vi "Modbus MFC Example.vi"() -> ()   [LabVIEW 2011]
doc: "This VI is an example program of how to use the MKS Modbus Drivers. This VI is only intended to demonstrate the drivers and is not meant to be used as a diagnostic tool."
uses:
  Type Definitions/Modbus Action.ctl
panel:
  out "Valve Drive(%)":sgl min=0 step=1 format="%.1f"
  out "MFC Info":T1
  in  "Flow Zero":bool
  in  "Valve Override":enum32{"Normal", "Close", "Open"}(radio)
  in  "Setpoint":dbl caption="Setpoint(sccm)" min=0.0 step=1.0 format="%#.6g"
  in  "Stop":bool
  in  "Close MB":bool
  in  "Initialize":bool
  in  "MFC IP Address":string="192.168.2.155"
  out "Waveform Chart":cluster{"Flow(sccm)":sgl, "Setpoint":sgl}(graph)
  # "Modbus MFC Example"
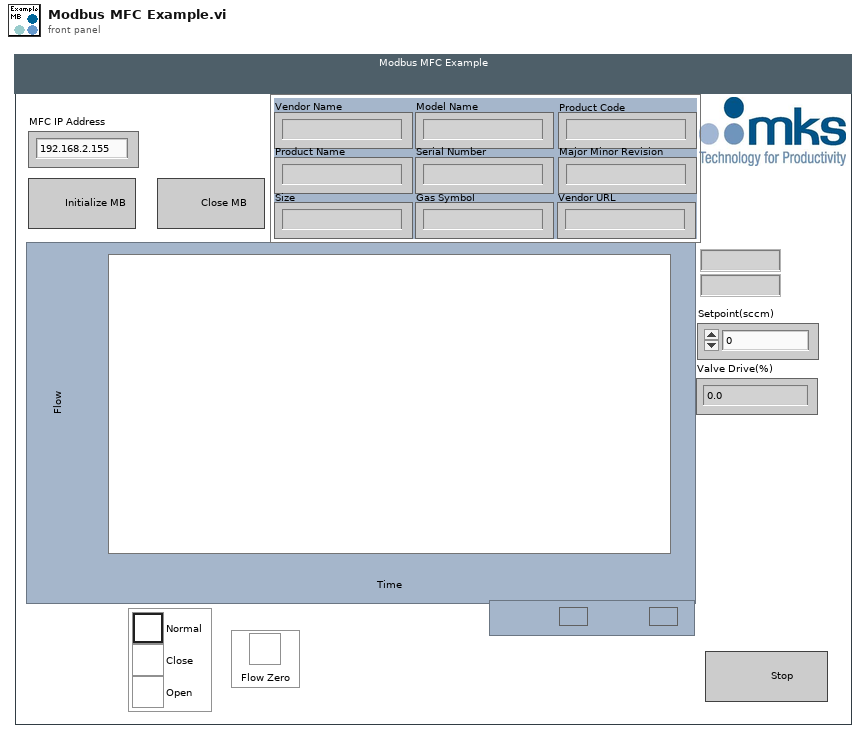
[diagram p1: front panel]
types:
  T1 = cluster{"Vendor Name":string, "Product Code":string, "Major Minor Revision":string, "Vendor URL":string, "Product Name":string, "Model Name":string, "Gas Symbol":string, "Serial Number":string, "Size":string}
  T2 = typedef "Modbus Action.ctl" = enum16{"Read", "Write"}
  T3 = enum8{"Enabled", "Disabled", "Disabled and Grayed Out"}
  T4 = typedef "Valve Override.ctl" = enum16{"Normal", "Close", "Open"}
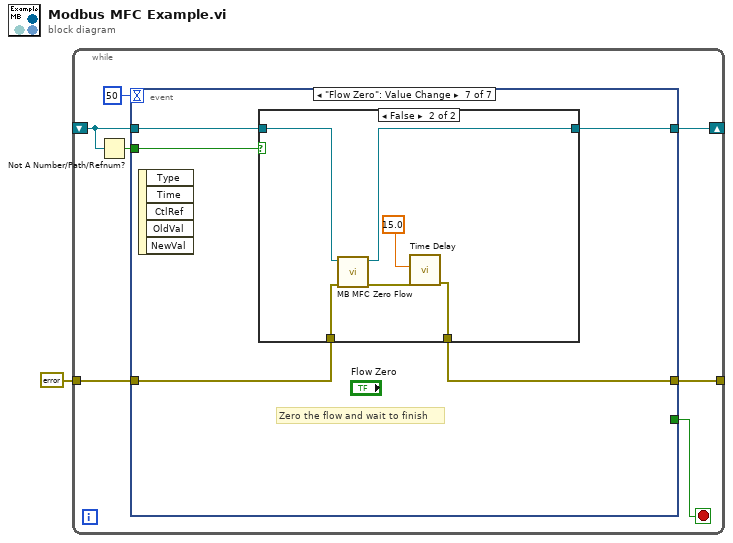
[diagram p0: block diagram]
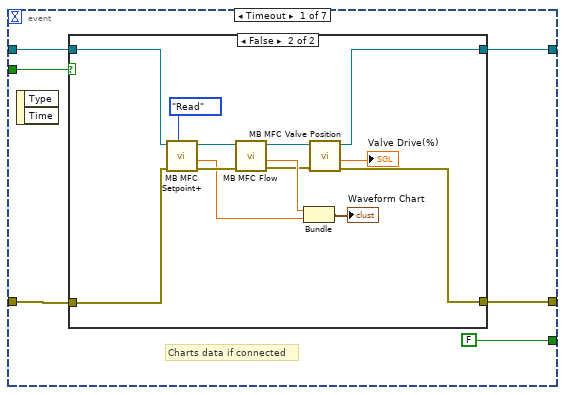
[diagram p2: hidden frame]
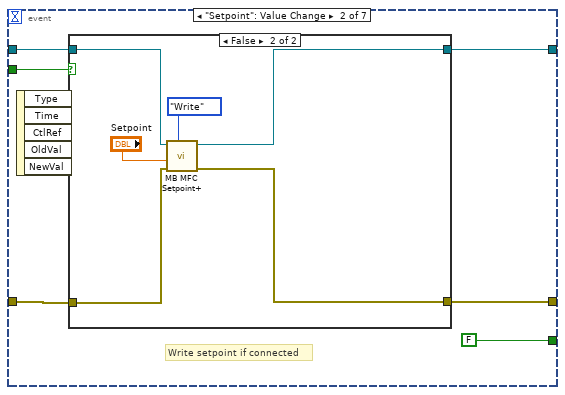
[diagram p4: hidden frame]
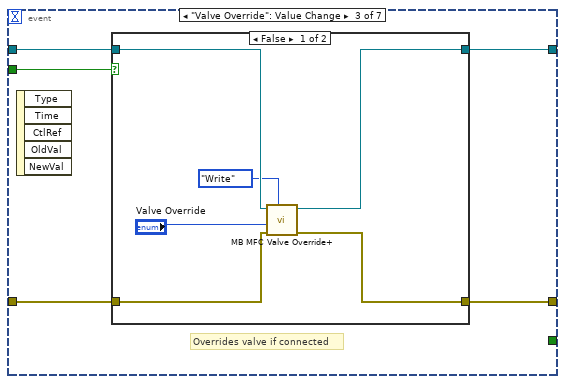
[diagram p6: hidden frame]
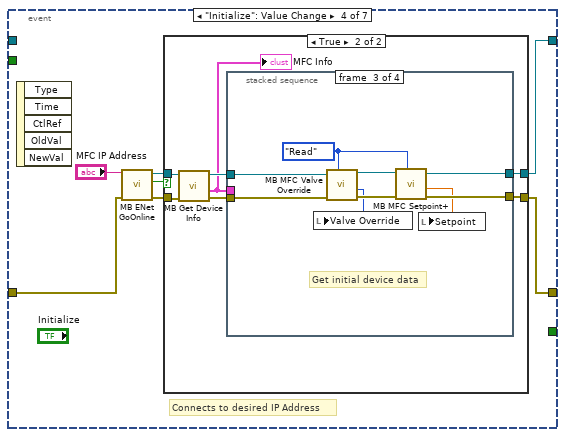
[diagram p8: hidden frame]
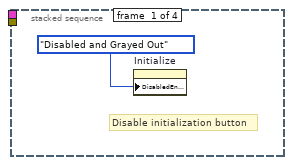
[diagram p10: hidden frame]
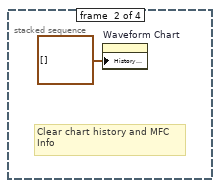
[diagram p11: hidden frame]
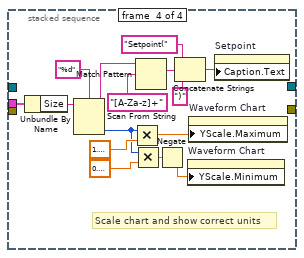
[diagram p12: hidden frame]
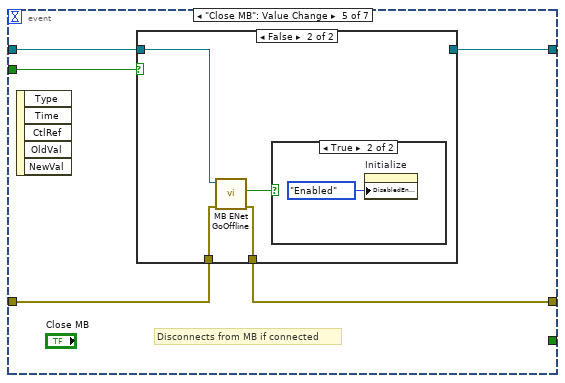
[diagram p13: hidden frame]
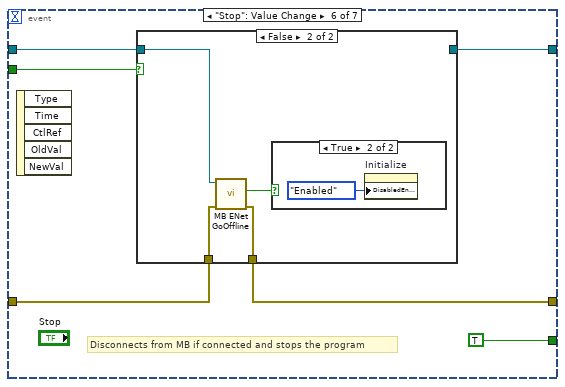
[diagram p16: hidden frame]
diagram:
  n1 = while {
    shift-right: [w6] -> _
    shift-left: _ -> [w3]
    tunnel: errorcluster {"status"=FALSE, "code"=0, "source"=""} ("error out") -> [w5]
    tunnel: [w4] -> _
    stop <- w7 stop-if-true
    n2 = Not A Number/Path/Refnum?(number/path/refnum=w3) -> (NaN/Path/Refnum?=w2:bool)
    n3 = event shown="[6] \"Flow Zero\": Value Change" {
      selector: _ -> [_ _ _ _ _ _ _]
      dyn-events: _ -> [_ _ _ _ _ _ _]
      timeout: 50 -> [_ _ _ _ _ _ _]
      tunnel: [FALSE FALSE _ _ _ TRUE _] -> w7
      tunnel: w3 -> [w10 w31 w48 _ w100 w113 w125]
      tunnel: [w11 w32 w47 w57 w99 w112 w124] -> w6
      tunnel: w5 -> [w13 w34 w45 w62 w102 w115 w127]
      tunnel: [w12 w33 w46 w58 w103 w116 w128] -> w4
      tunnel: w2 -> [w9 w30 w44 _ w101 w114 w126]
      event Timeout {
        # "Charts data if connected"
        n4 = event-data() -> ()  [unwired: 1 in, 2 out]
        n5 = case shown="False" w9 {
          tunnel: w10 -> [w16 w29]
          tunnel: w13 -> [w15 w27]
          tunnel: [w15 w18] -> w12
          tunnel: [w16 w20] -> w11
          frame True {
          }
          frame False {
            n6 = call "MB MFC Setpoint+.vi"("Action"=Modbus_Action."Read", "error in (no error)"=w27, "TCP Ref"=w29) -> ("error out"=w28:errorcluster, "Setpoint"=w24:sgl, "dup TCP Ref"=w26:refnum<k5>)  [unwired: 6 in]
            n7 = call "MB MFC Flow.vi"("error in (no error)"=w28, "TCP Ref"=w26) -> ("error out"=w19:errorcluster, "Flow(sccm)"=w25:sgl, "dup TCP Ref"=w21:refnum<k5>)  [unwired: 7 in]
            n8 = Bundle("Flow(sccm)"=w25, "Setpoint"=w24) -> (→"Waveform Chart":cluster{"Flow(sccm)":sgl, "Setpoint":sgl})  [unwired: 1 in]
            n9 = call "MB MFC Valve Position.vi"("error in (no error)"=w19, "TCP Ref"=w21) -> ("error out"=w18:errorcluster, "Valve Position(%)"=→"Valve Drive(%)":sgl, "dup TCP Ref"=w20:refnum<k5>)  [unwired: 7 in]
          }
        }
      }
      event "Setpoint": Value Change {
        # "Write setpoint if connected"
        n10 = event-data() -> ()  [unwired: 1 in, 5 out]
        n11 = case shown="False" w30 {
          tunnel: w31 -> [w37 w43]
          tunnel: w34 -> [w36 w42]
          tunnel: [w36 w38] -> w33
          tunnel: [w37 w39] -> w32
          frame True {
          }
          frame False {
            n12 = call "MB MFC Setpoint+.vi"("Action"=Modbus_Action."Write", "error in (no error)"=w42, "Setpoint"="Setpoint", "TCP Ref"=w43) -> ("error out"=w38:errorcluster, "dup TCP Ref"=w39:refnum<k5>)  [unwired: 5 in, 1 out]
          }
        }
      }
      event "Valve Override": Value Change {
        # "Overrides valve if connected"
        n13 = event-data() -> ()  [unwired: 1 in, 5 out]
        n14 = case shown="False" w44 {
          tunnel: w48 -> [w53 w55]
          tunnel: [w50 w55] -> w47
          tunnel: [w51 w56] -> w46
          tunnel: w45 -> [w54 w56]
          frame False {
            n15 = call "MB MFC Valve Override+.vi"("Action"=Modbus_Action."Write", "error in (no error)"=w54, "Override"="Valve Override", "TCP Ref"=w53) -> ("error out"=w51:errorcluster, "dup TCP Ref"=w50:refnum<k5>)  [unwired: 5 in, 1 out]
          }
          frame True {
          }
        }
      }
      event "Initialize": Value Change {
        # "Connects to desired IP Address"
        n16 = event-data() -> ()  [unwired: 1 in, 5 out]
        n17 = call "MB ENet GoOnline.vi"("error in (no error)"=w62, "IP Address"="MFC IP Address") -> ("error out"=w59:errorcluster, "OK"=w61:bool, "TCP Ref"=w60:refnum<k5>)  [unwired: 7 in]
        n18 = case shown="True" w61 {
          tunnel: w60 -> [w65 w70]
          tunnel: [w65 w67] -> w57
          tunnel: w59 -> [w64 w71]
          tunnel: [w64 w72] -> w58
          frame False {
          }
          frame True {
            n19 = call "MB Get Device Info.vi"("error in (no error)"=w71, "TCP Ref:ValBlock"=w70) -> ("error out"=w68:errorcluster, "MFC Info"=w66:T1, "dup TCP Ref:ValBlock"=w69:refnum<k5>)  [unwired: 7 in]
            "MFC Info" <- w66
            n20 = stacked-sequence {
              tunnel: [_ _ w83 _] -> w72
              tunnel: w69 -> [_ _ w78 _]
              tunnel: w68 -> [_ _ w77 _]
              tunnel: [_ _ w75 _] -> w67
              tunnel: w66 -> [_ _ _ w84]
              frame #0 {
                # "Disable initialization button"
                n21 = property on="Initialize" class="Bool"("DisabledEnum"=T3."Disabled and Grayed Out" ("Disabled")) -> ()  [unwired: 2 in, 2 out]
              }
              frame #1 {
                # "Clear chart history and MFC\nInfo"
                n22 = property on="Waveform Chart" class="WFChart (strict)"("History Data"=cluster{"Flow(sccm)":sgl, "Setpoint":sgl}[] []) -> ()  [unwired: 2 in, 2 out]
              }
              frame #2 {
                w80 = Modbus_Action."Read" ("Action")
                # "Get initial device data"
                n23 = call "MB MFC Valve Override.vi"("Action"=w80, "error in (no error)"=w77, "TCP Ref"=w78) -> ("error out"=w82:errorcluster, "Override"=w76:T4, "dup TCP Ref"=w81:refnum<k5>)  [unwired: 6 in]
                n24 = local write "Valve Override"(w76) -> ()
                n25 = call "MB MFC Setpoint+.vi"("Action"=w80, "error in (no error)"=w82, "TCP Ref"=w81) -> ("error out"=w83:errorcluster, "Setpoint"=w79:sgl, "dup TCP Ref"=w75:refnum<k5>)  [unwired: 6 in]
                n26 = local write "Setpoint"(w79) -> ()
              }
              frame #3 {
                # "Scale chart and show correct units"
                n27 = Unbundle By Name(w84) -> ("Size"=w97:string)
                n28 = Scan From String(format string="%d", input string=w97) -> (remaining string=w89:string, output 1=w92:i32)  [unwired: 3 in, 2 out]
                n29 = Multiply(x=w92, y=sgl 1.1) -> (x*y=w91:sgl)
                n30 = Multiply(x=w92, y=sgl 0.1) -> (x*y=w86:sgl)
                n31 = Match Pattern(string=w89, regular expression="[A-Za-z]+") -> (match substring=w88:string)  [unwired: 1 in, 3 out]
                n32 = Negate(x=w86) -> (-x=w85:sgl)
                n33 = Concatenate Strings("Setpoint(" ("string"), w88, ")" ("string")) -> (w94:string)
                n34 = property on="Waveform Chart" class="WFChart (strict)"("YScale.Minimum"=w85) -> ()  [unwired: 2 in, 2 out]
                n35 = property on="Waveform Chart" class="WFChart (strict)"("YScale.Maximum"=w91) -> ()  [unwired: 2 in, 2 out]
                n36 = property on="Setpoint" class="DigNum (strict)"("Caption.Text"=w94) -> ()  [unwired: 2 in, 2 out]
              }
            }
          }
        }
      }
      event "Close MB": Value Change {
        # "Disconnects from MB if connected"
        n37 = event-data() -> ()  [unwired: 1 in, 5 out]
        n38 = case shown="False" w101 {
          tunnel: [w104 w109] -> w103
          tunnel: w102 -> [w104 w108]
          tunnel: w100 -> [w105 w107]
          tunnel: [w105 _] -> w99
          frame True {
          }
          frame False {
            n39 = call "MB ENet GoOffline.vi"("error in (no error)"=w108, "TCP Ref:ValBlock"=w107) -> ("error out"=w109:errorcluster, "OK"=w106:bool)  [unwired: 7 in, 1 out]
            n40 = case shown="True" w106 {
              frame False {
              }
              frame True {
                n41 = property on="Initialize" class="Bool"("DisabledEnum"=T3."Enabled" ("Disabled")) -> ()  [unwired: 2 in, 2 out]
              }
            }
          }
        }
      }
      event "Stop": Value Change {
        # "Disconnects from MB if connected and stops the program"
        n42 = event-data() -> ()  [unwired: 1 in, 5 out]
        n43 = case shown="False" w114 {
          tunnel: [w117 w122] -> w116
          tunnel: w115 -> [w117 w121]
          tunnel: w113 -> [w118 w120]
          tunnel: [w118 _] -> w112
          frame True {
          }
          frame False {
            n44 = call "MB ENet GoOffline.vi"("error in (no error)"=w121, "TCP Ref:ValBlock"=w120) -> ("error out"=w122:errorcluster, "OK"=w119:bool)  [unwired: 7 in, 1 out]
            n45 = case shown="True" w119 {
              frame False {
              }
              frame True {
                n46 = property on="Initialize" class="Bool"("DisabledEnum"=T3."Enabled" ("Disabled")) -> ()  [unwired: 2 in, 2 out]
              }
            }
          }
        }
      }
      event "Flow Zero": Value Change {
        # "Zero the flow and wait to finish"
        n47 = event-data() -> ()  [unwired: 1 in, 5 out]
        n48 = case shown="False" w126 {
          tunnel: [w129 w131] -> w128
          tunnel: w127 -> [w129 w136]
          tunnel: w125 -> [w130 w135]
          tunnel: [w130 w133] -> w124
          frame True {
          }
          frame False {
            n49 = call "MB MFC Zero Flow.vi"("error in (no error)"=w136, "TCP Ref"=w135) -> ("error out"=w132:errorcluster, "dup TCP Ref"=w133:refnum<k5>)  [unwired: 8 in]
            n50 = call "Time Delay"("error in (no error)"=w132, "Delay Time (s)"=15.0) -> ("error out"=w131:errorcluster)  [unwired: 9 in]
          }
        }
      }
    }
  }
